vi "Array 2 Actuator Point.vi"(1 "Array":dbl[](array[numeric])) -> (0 "Actuator Point":T1)   [LabVIEW 2009]
uses:
  Metadata/Actuator Point.ctl
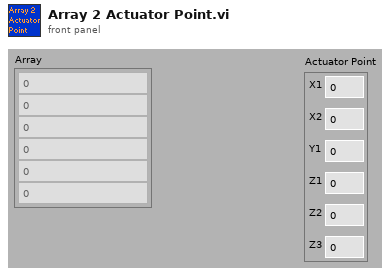
[diagram p1: front panel]
types:
  T1 = typedef "Actuator Point.ctl" = cluster{"X1":dbl, "X2":dbl, "Y1":dbl, "Z1":dbl, "Z2":dbl, "Z3":dbl}
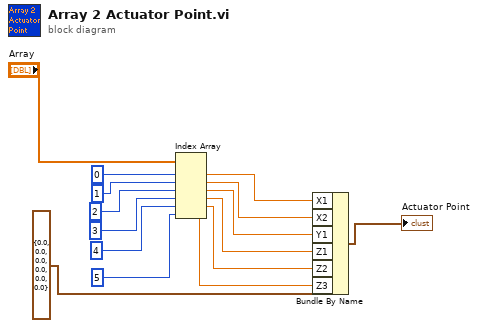
[diagram p0: block diagram]
diagram:
  n1 = Index Array(array="Array", index #1=0 ("index"), index #2=1 ("index"), index #3=2 ("index"), index #4=3 ("index"), index #5=4 ("index"), index #6=5 ("index")) -> (element #1=w8:dbl, element #2=w9:dbl, element #3=w10:dbl, element #4=w11:dbl, element #5=w12:dbl, element #6=w13:dbl)
  n2 = Bundle By Name(cluster=T1 {"X1"=0.0, "X2"=0.0, "Y1"=0.0, "Z1"=0.0, "Z2"=0.0, "Z3"=0.0} ("Actuator Point"), "X1"=w8, "X2"=w9, "Y1"=w10, "Z1"=w11, "Z2"=w12, "Z3"=w13) -> (→"Actuator Point":T1)
